vi "jsonKeys.vi"(8 "error in (no error)":errorcluster, 10 "path":string, 11 "d in":i64) -> (0 "error out":errorcluster, 2 "keys":string[](array[string]), 3 "d out":i64)   [LabVIEW 2015, in "rapidjson wrapper.lvlib"]
uses:
  rapidjson wrapper.lvlib
panel:
  out "return type":string
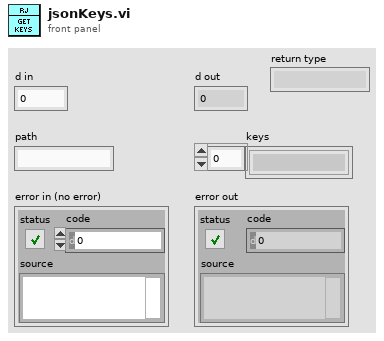
[diagram p1: front panel]
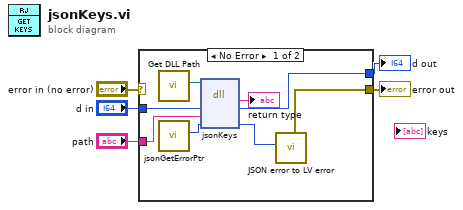
[diagram p0: block diagram]
diagram:
  n1 = case shown="No Error" "error in (no error)" {
    selector: "error in (no error)" -> [_ w15]
    tunnel: [w10 w15] -> w5
    tunnel: "d in" -> [w9 w14]
    tunnel: [w8 w14] -> w2
    tunnel: "path" -> [w7 _]
    frame No Error {
      n2 = call "Get DLL Path.vi"() -> ("Path"=w13:path)  [unwired: 11 in]
      n3 = call "jsonGetErrorPtr.vi"() -> ("return type"=w12:i64)  [unwired: 10 in, 1 out]
      n4 = dll-call lib="C:/Users/tblair/Documents/Git Projects/LVrapidjson core/lvrjs/Debug/lvrjs.dll" fn="jsonKeys"(path in=w13, "d"=w9, "path"=w7, "jsonError"=w12) -> ("return type"=→"return type":string, "d"=w8:i64, "jsonError"=w11:i64)  [unwired: 3 in, 2 out]
      n5 = call "JSON error to LV error.vi"("jsonError"=w11) -> ("error out"=w10:errorcluster)  [unwired: 10 in]
    }
    frame Error {
    }
  }
  "error out" <- w5
  "d out" <- w2
